vi "Vertically distribute controls from list.vi"(8 "error in":errorcluster, 9 "Ordered parent labels":string[](array[string]), 10 "Ordered item labels":string[](array[string]), 11 "Sorted control references in":refnum<vi>[](array[refnum])) -> (0 "error out":errorcluster, 3 "Sorted control references out":refnum<vi>[](array[refnum]))   [LabVIEW 2020, in "verticalDistribution.lvlib"]
uses:
  <vilib>/Utility/vertDist/verticalDistribution.lvlib
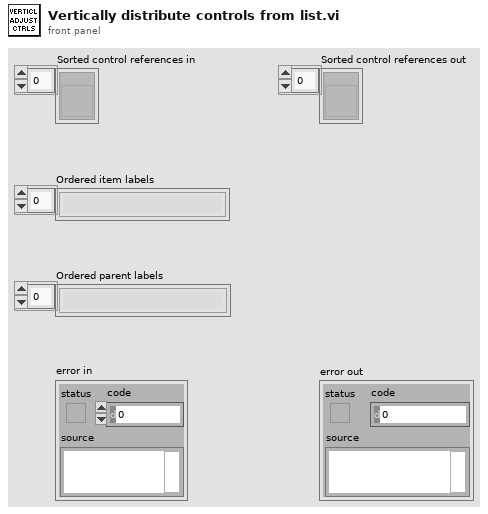
[diagram p1: front panel]
types:
  T1 = typedef "LVRectTypeDef.ctl" = cluster{"Left":i16, "Top":i16, "Right":i16, "Bottom":i16}
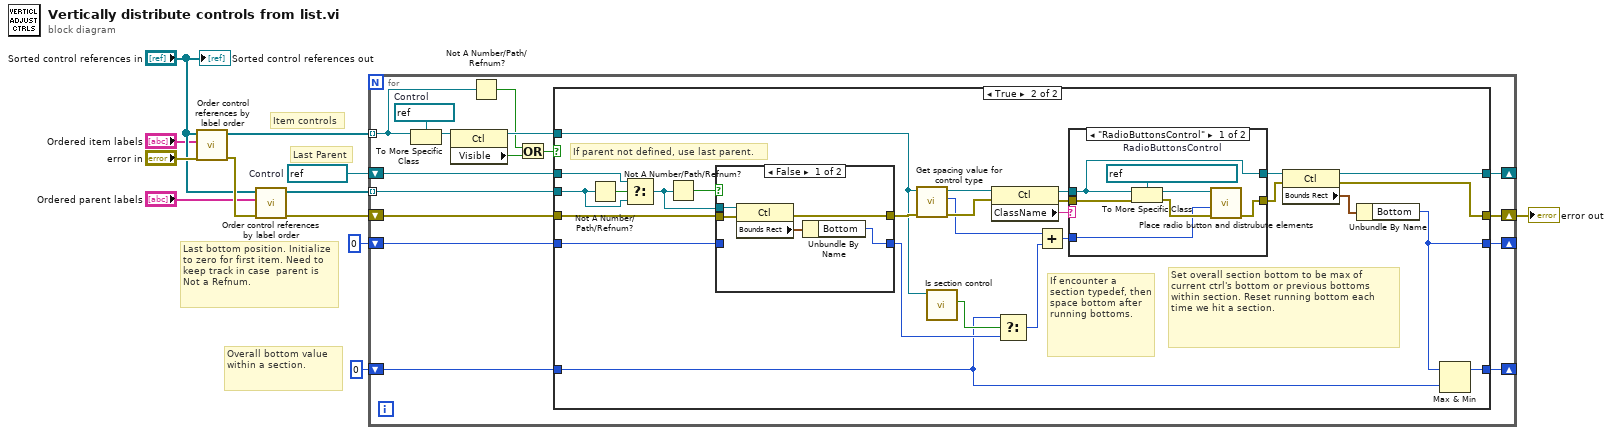
[diagram p0: block diagram]
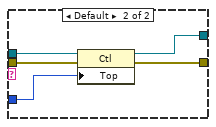
[diagram p4: hidden frame]
diagram:
  w8 = refnum<vi> refnum  # Control
  # "Item controls"
  # "Last Parent"
  # "Overall bottom value within a section."
  # "Last bottom position. Initialize to zero for first item. Need to keep track in case  parent is Not a Refnum."
  n1 = call <vilib>:"Order control references by label order.vi"("error in"="error in", "Ordered Labels"="Ordered item labels", "Control References"="Sorted control references in") -> ("error out"=w12:errorcluster, "Ordered control references"=w6:refnum<vi>[])  [unwired: 7 out]
  n2 = call <vilib>:"Order control references by label order.vi"("error in"=w12, "Ordered Labels"="Ordered parent labels", "Control References"="Sorted control references in") -> ("error out"=w11:errorcluster, "Ordered control references"=w7:refnum<vi>[])  [unwired: 7 out]
  n3 = for {
    tunnel: w6 -> [w20] mode=indexing
    tunnel: w7 -> [w25] mode=indexing
    shift-right: [w27] -> w9
    shift-left: w11 -> [w28]
    shift-right: [w24] -> _
    shift-left: w8 -> [w26]
    shift-right: [w15] -> _
    shift-left: i16 0 ("bottom") -> [w16]
    shift-right: [w13] -> _
    shift-left: i16 0 ("bottom") -> [w14]
    w22 = refnum<vi> refnum  # Control
    n4 = To More Specific Class(target class=w22, reference=w20) -> (specific class reference=w23:refnum<vi>)  [unwired: 1 in, 1 out]
    n5 = property class="Ctl"(reference=w23) -> (reference out=w21:refnum<vi>, "Visible"=w17:bool)  [unwired: 1 in, 1 out]
    n6 = Not A Number/Path/Refnum?(number/path/refnum=w20) -> (NaN/Path/Refnum?=w18:bool)
    n7 = Or(x=w18, y=w17) -> (x .or. y?=w19:bool)
    n8 = case shown="True" w19 {
      tunnel: w28 -> [w32 w59]
      tunnel: [w32 w54] -> w27
      tunnel: w26 -> [w31 w52]
      tunnel: w25 -> [_ w51]
      tunnel: [w31 w38] -> w24
      tunnel: w21 -> [_ w42]
      tunnel: w16 -> [w30 w44]
      tunnel: [w30 w36] -> w15
      tunnel: w14 -> [w29 w34]
      tunnel: [w29 w33] -> w13
      frame False {
        # "If control is not visible or control reference is Not a Refnum, then skip it.  Don't update the control in shift register."
      }
      frame True {
        # "Set overall section bottom to be max of current ctrl's bottom or previous bottoms\nwithin section. Reset running bottom each time we hit a section."
        # "If encounter a section typedef, then space bottom after running bottoms."
        # "If parent not defined, use last parent."
        n9 = Not A Number/Path/Refnum?(number/path/refnum=w51) -> (NaN/Path/Refnum?=w53:bool)
        n10 = Select(t=w52, s=w53, f=w51) -> (s? t:f=w43:refnum<vi>)
        n11 = Not A Number/Path/Refnum?(number/path/refnum=w43) -> (NaN/Path/Refnum?=w50:bool)
        n12 = case shown="False" w50 {
          tunnel: w59 -> [w64 w66]
          tunnel: [w62 w65] -> w37
          tunnel: [w63 w66] -> w58
          tunnel: w43 -> [w60 _]
          tunnel: w44 -> [_ w65]
          frame False {
            n13 = property class="Ctl"(reference=w60, error in=w64) -> (error out=w63:errorcluster, "Bounds Rect"=w61:T1)  [unwired: 1 out]
            n14 = Unbundle By Name(w61) -> ("Bottom"=w62:i16)
          }
          frame True {
            # "First item or parent is Not a Refnum"
          }
        }
        n15 = call <vilib>:"Get spacing value for control type.vi"("error in"=w58, "control reference in"=w42) -> ("error out"=w57:errorcluster, "Spacing value"=w45:u32, "control reference out"=w47:refnum<vi>)  [unwired: 7 out]
        n16 = call <vilib>:"Is section control.vi"("control reference in"=w42) -> ("Section"=w35:bool)  [unwired: 1 in, 9 out]
        n17 = property class="Ctl"(reference=w47, error in=w57) -> (reference out=w46:refnum<vi>, error out=w56:errorcluster, "ClassName"=w49:string)
        n18 = Select(t=w34, s=w35, f=w37) -> (s? t:f=w41:i16)
        n19 = Add(x=w45, y=w41) -> (x+y=w48:u32)
        n20 = case shown="\"RadioButtonsControl\"" w49 {
          tunnel: [w73 w78] -> w55
          tunnel: w48 -> [w70 w75]
          tunnel: w56 -> [w72 w77]
          tunnel: w46 -> [w67 w76]
          tunnel: [w67 w74] -> w40
          frame "RadioButtonsControl" {
            w69 = refnum<vi> refnum  # RadioButtonsControl
            n21 = To More Specific Class(target class=w69, reference=w67, error in=w72) -> (specific class reference=w68:refnum<vi>, error out=w71:errorcluster)
            n22 = call <vilib>:"Place radio button and distrubute elements.vi"("error in"=w71, "Bottom of last control"=w70, "radio button reference"=w68) -> ("error out"=w73:errorcluster)  [unwired: 8 out]
          }
          frame Default {
            n23 = property class="Ctl"(reference=w76, error in=w77, "Top"=w75) -> (reference out=w74:refnum<vi>, error out=w78:errorcluster)
          }
        }
        n24 = property class="Ctl"(reference=w40, error in=w55) -> (reference out=w38:refnum<vi>, error out=w54:errorcluster, "Bounds Rect"=w39:T1)
        n25 = Unbundle By Name(w39) -> ("Bottom"=w36:i16)
        n26 = Max & Min(x=w36, y=w34) -> (max(x,y)=w33:i16)  [unwired: 1 out]
      }
    }
  }
  "error out" <- w9
  "Sorted control references out" <- "Sorted control references in"
